vi "HRTF-About Box.vi"() -> ()   [LabVIEW 2015]
uses:
  <resource>/objmgr/daqmx.rc
panel:
  out "Version":string
  in  "OK":bool
  # "HRTF Measurement"
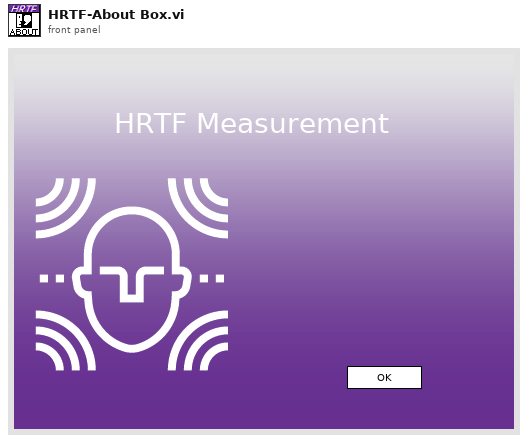
[diagram p1: front panel]
types:
  T1 = cluster{"Major":i32, "Minor":i32, "Build":i32, "Private":i32, "FileVersion":string, "ProductName":string, "InternalName":string, "CompanyName":string, "LegalCopyright":string, "FileDescription":string}
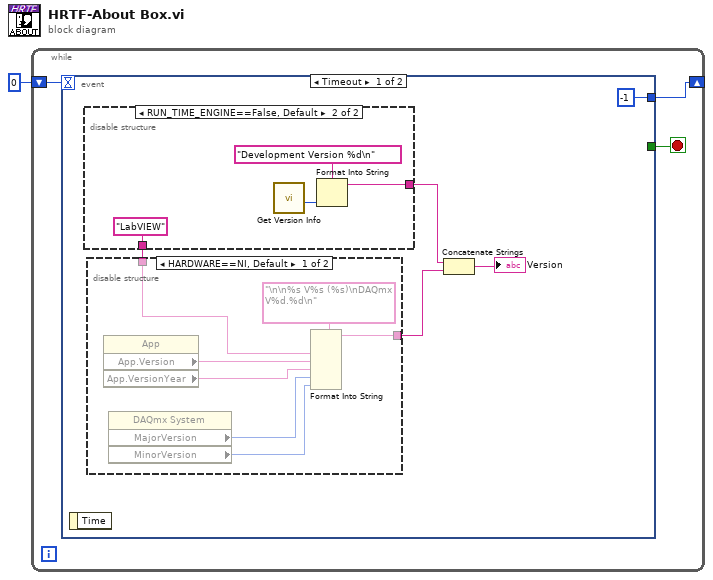
[diagram p0: block diagram]
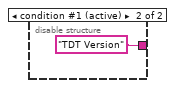
[diagram p2: hidden frame]
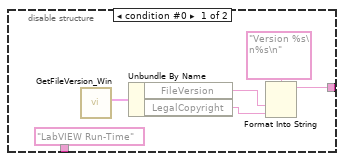
[diagram p3: hidden frame]
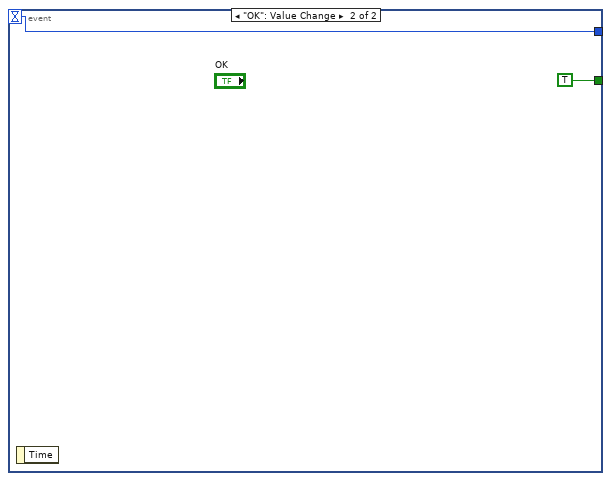
[diagram p4: hidden frame]
diagram:
  n1 = while {
    shift-right: [w2] -> _
    shift-left: 0 -> [w3]
    stop <- w4 stop-if-true
    n2 = event shown="[0] Timeout" {
      selector: _ -> [_ _]
      dyn-events: _ -> [_ _]
      timeout: w3 -> [_ w28]
      tunnel: [_ TRUE] -> w4
      tunnel: [-1 w28] -> w2
      event Timeout {
        n3 = event-data() -> ()  [unwired: 1 in, 1 out]
        n4 = disable-structure shown="RUN_TIME_ENGINE==False, Default" {
          disable-tunnel: [w21 w25] -> w8
          disable-tunnel: ["LabVIEW Run-Time" "LabVIEW"] -> w5
          frame condition #0 {
            n5 = call "GetFileVersion_Win.vi"() -> ("File Info Out"=w22:T1)  [unwired: 9 in, 2 out]
            n6 = Unbundle By Name(w22) -> ("FileVersion"=w20:string, "LegalCopyright"=w19:string)
            n7 = Format Into String(format string="Version %s\n%s\n", w20, w19) -> (resulting string=w21:string)  [unwired: 2 in, 1 out]
          }
          frame condition #1 (active) {
            n8 = call "Get Version Info.vi"() -> ("Expt VIs Version out"=w26:i32)  [unwired: 10 in, 1 out]
            n9 = Format Into String(format string="Development Version %d\n" ("PF Version"), w26) -> (resulting string=w25:string)  [unwired: 2 in, 1 out]
          }
        }
        n10 = disable-structure shown="HARDWARE==NI, Default" {
          disable-tunnel: [w12 "TDT Version"] -> w6
          disable-tunnel: w5 -> [w13 _]
          frame condition #0 {
            n11 = property class="App"() -> ("App.Version"=w15:string, "App.VersionYear"=w14:string)  [unwired: 2 in, 2 out]
            n12 = property class="DAQmx System"() -> ("MajorVersion"=w11:u32, "MinorVersion"=w10:u32)  [unwired: 2 in, 2 out]
            n13 = Format Into String(format string="\n\n%s V%s (%s)\nDAQmx V%d.%d\n", w13, w15, w14, w11, w10) -> (resulting string=w12:string)  [unwired: 2 in, 1 out]
          }
          frame condition #1 (active) {
          }
        }
        n14 = Concatenate Strings(w8, w6) -> (→"Version":string)
      }
      event "OK": Value Change {
        n15 = event-data() -> ()  [unwired: 1 in, 1 out]
      }
    }
  }
